vi "SpecAn Configure IM.vi"(0 "Instrument Handle In":refnum<k21>, 1 "Selector String":string, 5 "IM Config":T1={"Maximum Intermod Order"=3, "Lower Tone Frequency (Hz)"=-1000000.0, "Upper Tone Frequency (Hz)"=1000000.0, "Measurement Method"=0, "Averaging Count"=10, "Averaging Enabled"=0, "Averaging Type"=0, "Sweep Time Interval (s)"=0.001, "Sweep Time Auto"=1, "RBW Filter Type"=1, "RBW (Hz)"=10000.0, "RBW Auto"=1} {"RBW Auto" items=["False", "True"]; "RBW (Hz)" format="%.3p"; "RBW Filter Type" items=["FFT Based", "Gaussian", "Flat"]; "Sweep Time Auto" items=["False", "True"]; "Sweep Time Interval (s)" format="%.2p"; "Averaging Type" items=["RMS", "Log", "Scalar", "Max", "Min"]; "Averaging Enabled" items=["False", "True"]; "Measurement Method" items=["Normal", "Dynamic Range", "Segmented"]; "Upper Tone Frequency (Hz)" format="%.3p"; "Lower Tone Frequency (Hz)" format="%.3p"; "Maximum Intermod Order" items=["3"=3, "5"=5, "7"=7, "9"=9]}, 11 "error in (no error)":errorcluster) -> (4 "Instrument Handle Out":refnum<k21>, 15 "error out":errorcluster)   [LabVIEW 2016, in "RFmxSpecAn.lvlib"]
doc: "Configures common settings for the IM measurement and selects the measurement."
uses:
  RFmxSpecAn.lvlib
  SpecAn IM Configuration.ctl
  <vilib>/RFmx/SpecAn/mx/RFmxSpecAn.llb/RFmxSpecAn Select Measurement (Single).vi
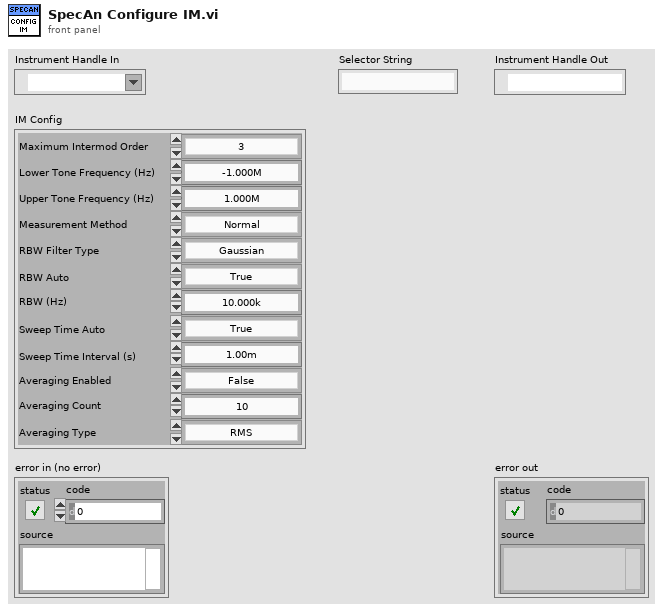
[diagram p1: front panel]
types:
  T1 = typedef "RFmxSpecAn.lvlib/SpecAn IM Configuration.ctl" = cluster{"Maximum Intermod Order":i32, "Lower Tone Frequency (Hz)":dbl, "Upper Tone Frequency (Hz)":dbl, "Measurement Method":i32, "Averaging Count":i32, "Averaging Enabled":i32, "Averaging Type":i32, "Sweep Time Interval (s)":dbl, "Sweep Time Auto":i32, "RBW Filter Type":i32, "RBW (Hz)":dbl, "RBW Auto":i32}
  T2 = enum16{"ACP", "CCDF", "CHP", "FCnt", "Harmonics", "OBW", "SEM", "Spectrum", "Spur", "TXP", "AMPM", "DPD", "IQ", "IM", "NF", "PhaseNoise", "PAVT"}
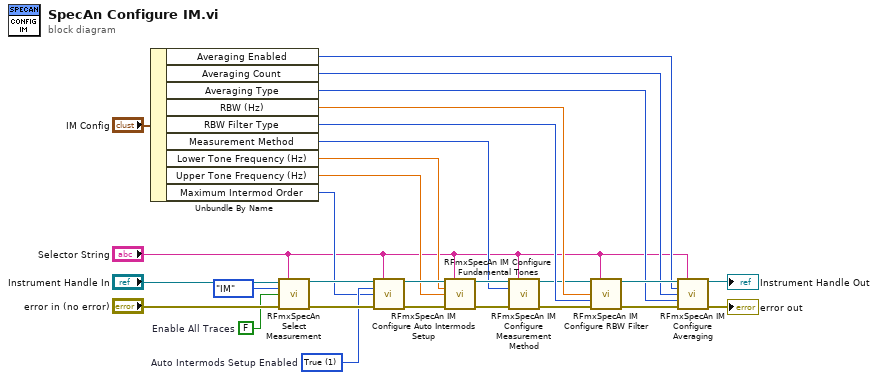
[diagram p0: block diagram]
diagram:
  w11 = 1 items=["False", "True"]  # Auto Intermods Setup Enabled
  w13 = FALSE  # Enable All Traces
  n1 = Unbundle By Name("IM Config") -> ("Averaging Enabled"=w16:i32, "Averaging Count"=w17:i32, "Averaging Type"=w18:i32, "RBW (Hz)"=w19:dbl, "RBW Filter Type"=w20:i32, "Measurement Method"=w2:i32, "Lower Tone Frequency (Hz)"=w7:dbl, "Upper Tone Frequency (Hz)"=w6:dbl, "Maximum Intermod Order"=w10:i32)
  n2 = call-poly <vilib>:"RFmxSpecAn Select Measurement.vi"("Instrument Handle In"="Instrument Handle In", "Selector String"="Selector String", "Measurement"=T2."IM", "Enable All Traces"=w13, "error in (no error)"="error in (no error)") -> ("Instrument Handle Out"=w21:refnum<k21>, "error out"=w28:errorcluster)  [unwired: 9 in]
  n3 = call <vilib>:"RFmxSpecAn IM Configure Auto Intermods Setup.vi"("Instrument Handle In"=w21, "Selector String"="Selector String", "Auto Intermods Setup Enabled"=w11, "Maximum Intermod Order"=w10, "error in (no error)"=w28) -> ("Instrument Handle Out"=w8:refnum<k21>, "error out"=w27:errorcluster)  [unwired: 9 in]
  n4 = call <vilib>:"RFmxSpecAn IM Configure Fundamental Tones.vi"("Instrument Handle In"=w8, "Selector String"="Selector String", "Lower Tone Frequency (Hz)"=w7, "Upper Tone Frequency (Hz)"=w6, "error in (no error)"=w27) -> ("Instrument Handle Out"=w4:refnum<k21>, "error out"=w9:errorcluster)  [unwired: 9 in]
  n5 = call <vilib>:"RFmxSpecAn IM Configure Measurement Method.vi"("Instrument Handle In"=w4, "Selector String"="Selector String", "Measurement Method"=w2, "error in (no error)"=w9) -> ("Instrument Handle Out"=w3:refnum<k21>, "error out"=w5:errorcluster)  [unwired: 10 in]
  n6 = call <vilib>:"RFmxSpecAn IM Configure RBW Filter.vi"("Instrument Handle In"=w3, "Selector String"="Selector String", "RBW (Hz)"=w19, "RBW Filter Type"=w20, "error in (no error)"=w5) -> ("Instrument Handle Out"=w25:refnum<k21>, "error out"=w26:errorcluster)  [unwired: 9 in]
  n7 = call <vilib>:"RFmxSpecAn IM Configure Averaging.vi"("Instrument Handle In"=w25, "Selector String"="Selector String", "Averaging Enabled"=w16, "Averaging Count"=w17, "Averaging Type"=w18, "error in (no error)"=w26) -> ("Instrument Handle Out"=→"Instrument Handle Out":refnum<k21>, "error out"=→"error out":errorcluster)  [unwired: 8 in]
